vi "Register gRPC Methods.vi"(8 "error in (no error)":errorcluster, 11 "Template Server in":refnum<class "GreeterService.lvclass">) -> (0 "error out":errorcluster, 3 "Template Server out":refnum<class "GreeterService.lvclass">)   [LabVIEW 2019, in "Generated_server.lvlib" / "GreeterService.lvclass"]
uses:
  GreeterService.lvclass
  typeDefs/Server Internal UEs.ctl
  typeDefs/Server Internal Message.ctl
  typeDefs/Server gRPC UEs.ctl
  <vilib>/gRPC/LabVIEW gRPC Library/Server API/typeDefs/gRPCId Cluster.ctl
  <vilib>/gRPC/LabVIEW gRPC Library/Shared/grpcId.ctl
  GreeterService.lvclass/GreeterService.ctl
  <vilib>/gRPC/LabVIEW gRPC Library/grpc-lvsupport-release.lvlib
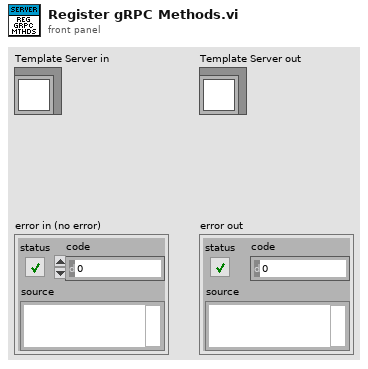
[diagram p1: front panel]
types:
  T1 = typedef "Generated_server.lvlib/GreeterService.lvclass/Server gRPC UEs.ctl" = cluster{"GreeterService UnaryMethod gRPC UE":refnum<user-event>, "GreeterService ServerStreamingMethod gRPC UE":refnum<user-event>, "GreeterService ClientStreamingMethod gRPC UE":refnum<user-event>, "GreeterService BidirectionalStreamingMethod gRPC UE":refnum<user-event>}
  T2 = typedef "Generated_server.lvlib/GreeterService.lvclass/Server Internal UEs.ctl" = cluster{"GreeterService UnaryMethod Internal UE":refnum<user-event>, "GreeterService ServerStreamingMethod Internal UE":refnum<user-event>, "GreeterService ClientStreamingMethod Internal UE":refnum<user-event>, "GreeterService BidirectionalStreamingMethod Internal UE":refnum<user-event>}
  T3 = typedef "grpc-lvsupport-release.lvlib/grpcId.ctl" = u64
  T4 = typedef "Generated_server.lvlib/GreeterService.lvclass/Server Internal Message UE.ctl" = refnum<user-event>
  T5 = typedef "grpc-lvsupport-release.lvlib/gRPCId Cluster UE.ctl" = refnum<user-event>
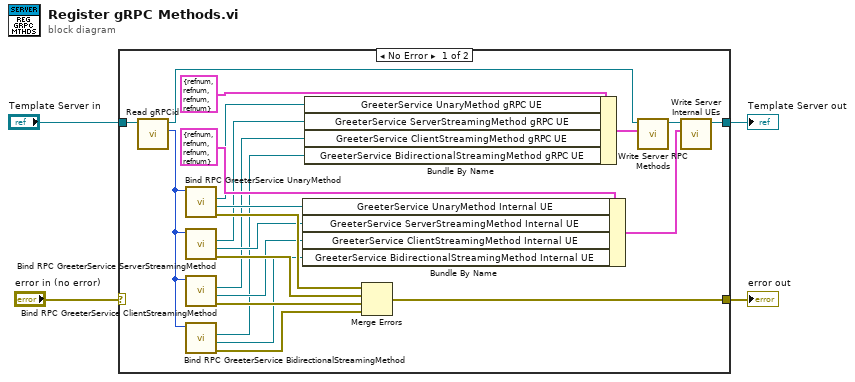
[diagram p0: block diagram]
diagram:
  n1 = case shown="No Error" "error in (no error)" {
    selector: "error in (no error)" -> [_ w27]
    tunnel: "Template Server in" -> [w18 w28]
    tunnel: [w26 w27] -> w3
    tunnel: [w25 w28] -> w2
    frame No Error {
      n2 = call-dynamic "Read gRPCid.vi"("iService in"=w18) -> ("gRPCid"=w17:T3, "iService out"=w19:refnum<class "GreeterService.lvclass">)  [unwired: 8 in, 1 out]
      n3 = call "Bind RPC GreeterService UnaryMethod.vi"("gRPCid server in"=w17) -> ("error out"=w16:errorcluster, "GreeterService UnaryMethod Internal UE"=w14:T4, "GreeterService UnaryMethod gRPC UE"=w15:T5)  [unwired: 7 in, 1 out]
      n4 = call "Bind RPC GreeterService ServerStreamingMethod.vi"("gRPCid server in"=w17) -> ("error out"=w13:errorcluster, "GreeterService ServerStreamingMethod Internal UE"=w11:T4, "GreeterService ServerStreamingMethod gRPC UE"=w12:T5)  [unwired: 7 in, 1 out]
      n5 = call "Bind RPC GreeterService ClientStreamingMethod.vi"("gRPCid server in"=w17) -> ("error out"=w10:errorcluster, "GreeterService ClientStreamingMethod Internal UE"=w8:T4, "GreeterService ClientStreamingMethod gRPC UE"=w9:T5)  [unwired: 7 in, 1 out]
      n6 = call "Bind RPC GreeterService BidirectionalStreamingMethod.vi"("gRPCid server in"=w17) -> ("error out"=w7:errorcluster, "GreeterService BidirectionalStreamingMethod Internal UE"=w5:T4, "GreeterService BidirectionalStreamingMethod gRPC UE"=w6:T5)  [unwired: 7 in, 1 out]
      n7 = Bundle By Name ("Bundle Internal UEs")(cluster=T2 {"GreeterService UnaryMethod Internal UE"=refnum, "GreeterService ServerStreamingMethod Internal UE"=refnum, "GreeterService ClientStreamingMethod Internal UE"=refnum, "GreeterService BidirectionalStreamingMethod Internal UE"=refnum} ("Server Internal UEs"), "GreeterService UnaryMethod Internal UE"=w14, "GreeterService ServerStreamingMethod Internal UE"=w11, "GreeterService ClientStreamingMethod Internal UE"=w8, "GreeterService BidirectionalStreamingMethod Internal UE"=w5) -> (w24:T2)
      n8 = Bundle By Name ("Bundle gRPC UEs")(cluster=T1 {"GreeterService UnaryMethod gRPC UE"=refnum, "GreeterService ServerStreamingMethod gRPC UE"=refnum, "GreeterService ClientStreamingMethod gRPC UE"=refnum, "GreeterService BidirectionalStreamingMethod gRPC UE"=refnum} ("gRPC Server Method Events"), "GreeterService UnaryMethod gRPC UE"=w15, "GreeterService ServerStreamingMethod gRPC UE"=w12, "GreeterService ClientStreamingMethod gRPC UE"=w9, "GreeterService BidirectionalStreamingMethod gRPC UE"=w6) -> (w21:T1)
      n9 = Merge Errors(w16, w13, w10, w7) -> (w26:errorcluster)
      n10 = call "Write Server RPC Methods.vi"("Server RPC Methods"=w21, "SignalGeneratorService in"=w19) -> ("SignalGeneratorService out"=w22:refnum<class "GreeterService.lvclass">)  [unwired: 8 in, 1 out]
      n11 = call "Write Server Internal UEs.vi"("Server Internal UEs"=w24, "SignalGeneratorService in"=w22) -> ("SignalGeneratorService out"=w25:refnum<class "GreeterService.lvclass">)  [unwired: 8 in, 1 out]
    }
    frame Error {
    }
  }
  "error out" <- w3
  "Template Server out" <- w2
